vi "EtherCAT_to_EtherNET.vi"() -> ()   [LabVIEW 2018]
uses:
  <resource>/objmgr/IndComECAT.rc
panel:
  out "Abort Code":u32
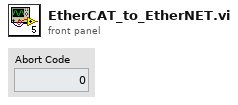
[diagram p1: front panel]
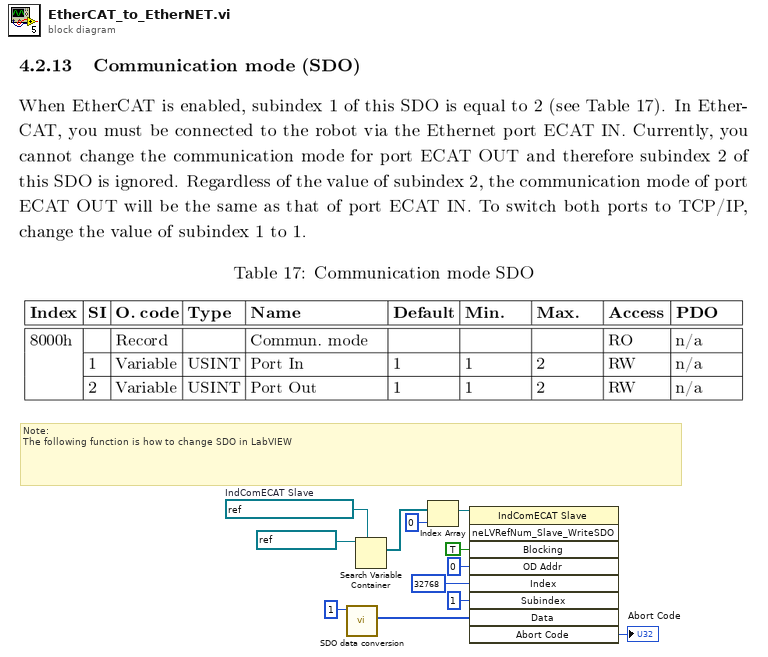
[diagram p0: block diagram]
diagram:
  w5 = refnum<k21> refnum  # IndComECAT Slave
  # "Note:\nThe following function is how to change SDO in LabVIEW"
  n1 = call "SDO data conversion.vi"("Decimal Input"=1) -> ("Array"=w3:u8[])  [unwired: 9 in, 1 out]
  n2 = Search Variable Container(7:w5, 11:refnum<k21> "ni.var.io:/" ("container refnum in")) -> (2:w7:refnum<k21>[])  [unwired: 4 in, 2 out]
  n3 = Index Array(array=w7, index=0) -> (element=w6:refnum<k21>)
  n4 = invoke class="IndComECAT Slave" method="neLVRefNum_Slave_WriteSDO"(reference=w6, "Blocking"=TRUE, "OD Addr"=u16 0, "Index"=u16 32768, "Subindex"=u8 1, "Data"=w3) -> ("Abort Code"=→"Abort Code":u32)  [unwired: 3 in, 8 out]
